vi "TxRx.vi"(5 "Reply Timeout Ms":i32=1000, 6 "Queue Name":string="firmata-serial-communication", 7 "Wait For Reply?":bool=TRUE, 8 "error in":errorcluster, 10 "Message":u8[](array[numeric]), 11 "Command":T1=enum."Transmit - Receive") -> (0 "error out":errorcluster, 2 "Reply":u8[](array[numeric]) format="%.0x")   [LabVIEW 2020, in "FirmataClient.lvlib"]
doc: "Obtains the communication links used to send and receive command and messages to and from the currently running trasnport engine. Note that these are \"named\" communication links. The name of Queue must match the name of the queue the Engine is servicing."
uses:
  Transports/Controls/Transport Commands.ctl
  Transports/Controls/Transport Queue Message.ctl
  Transports/Controls/Transport Notifier Response.ctl
  FirmataClient.lvlib
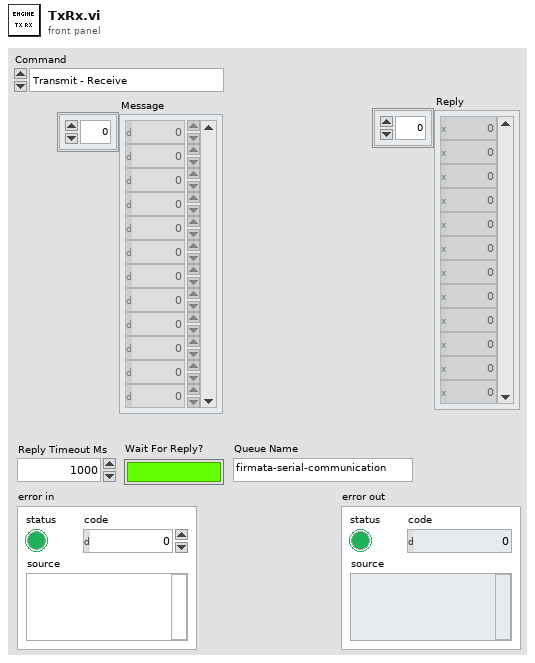
[diagram p1: front panel]
types:
  T1 = typedef "Transport Commands.ctl" = enum16{"Initialize", "Transmit - Receive", "Cleanup", "Cleanup And Stop"}
  T2 = typedef "Transport Queue Message.ctl" = cluster{"Command":T1, "Message":u8[]}
  T3 = typedef "Transport Notifier Response.ctl" = cluster{"Message":u8[], "Error":errorcluster}
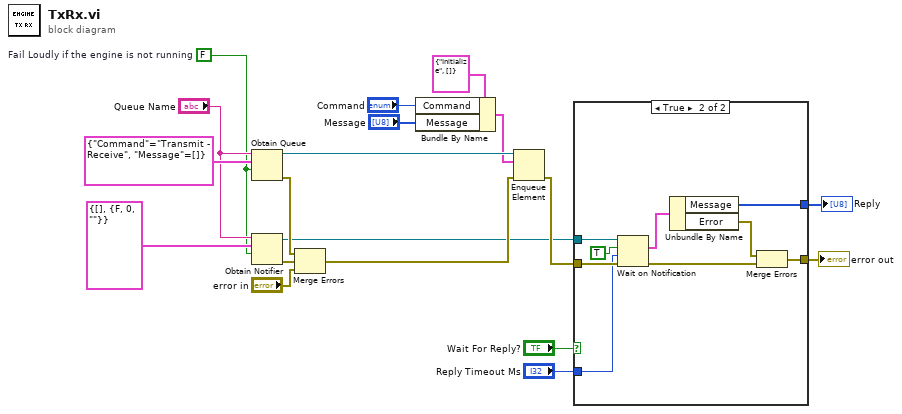
[diagram p0: block diagram]
diagram:
  w13 = FALSE  # Fail Loudly if the engine is not running
  n1 = Obtain Queue(name (unnamed)="Queue Name", element data type=T2 {"Command"=enum."Transmit - Receive", "Message"=[]} ("Transport Qiueue Message"), create if not found? (T)=w13) -> (queue out=w11:refnum<queue>, error out=w16:errorcluster)  [unwired: 2 in, 1 out]
  n2 = Obtain Notifier(name (unnamed)="Queue Name", notification data type=T3 {"Message"=[], "Error"={"status"=FALSE, "code"=0, "source"=""}} ("Transport Notifier Response"), create if not found? (T)=w13) -> (notifier out=w9:refnum<notifier>, error out=w15:errorcluster)  [unwired: 1 in, 1 out]
  n3 = Merge Errors(w16, w15, "error in") -> (w10:errorcluster)
  n4 = Bundle By Name(cluster=T2 {"Command"=enum."Initialize", "Message"=[]} ("element"), "Command"="Command", "Message"="Message") -> (w3:T2)
  n5 = Enqueue Element(queue=w11, element=w3, error in (no error)=w10) -> (error out=w12:errorcluster)  [unwired: 1 in, 2 out]
  n6 = case shown="True" "Wait For Reply?" {
    tunnel: w12 -> [w20 w28]
    tunnel: w9 -> [_ w27]
    tunnel: [w20 w23] -> w8
    tunnel: [_ w22] -> w7
    tunnel: "Reply Timeout Ms" -> [_ w21]
    frame False {
    }
    frame True {
      n7 = Wait on Notification(notifier=w27, ignore previous (F)=TRUE, timeout in ms (-1)=w21, error in (no error)=w28) -> (notification=w26:T3, error out=w24:errorcluster)  [unwired: 2 out]
      n8 = Unbundle By Name(w26) -> ("Message"=w22:u8[], "Error"=w25:errorcluster)
      n9 = Merge Errors(w25, w24) -> (w23:errorcluster)
    }
  }
  "error out" <- w8
  "Reply" <- w7
